vi "Drive Toggle 2016.vi"(10 "# of cases":i32=2, 11 "Toggle":bool) -> (3 "mode switch":i32)   [LabVIEW 2015]
uses:
  <vilib>/ptbypt/NI_PtbyPt.lvlib
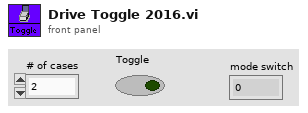
[diagram p1: front panel]
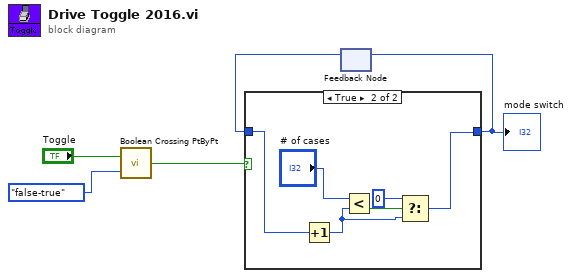
[diagram p0: block diagram]
diagram:
  n1 = call <vilib>:"Boolean Crossing PtByPt.vi"("direction"=enum16{"either", "false-true", "true-false"}."false-true", "input"="Toggle") -> ("crossing"=w3:bool)  [unwired: 1 in]
  n2 = feedback #1() -> (w1:i32)  [unwired: 1 in]
  n3 = case shown="True" w3 {
    tunnel: [w6 w9] -> w2
    tunnel: w1 -> [w6 w7]
    frame False {
    }
    frame True {
      n4 = Increment(x=w7) -> (x+1=w8:i32)
      n5 = Less?(x="# of cases", y=w8) -> (x < y?=w11:bool)
      n6 = Select(t=0, s=w11, f=w8) -> (s? t:f=w9:i32)
    }
  }
  "mode switch" <- w2
  n7 = feedback-in #1(w2) -> ()
